vi "Calculate_Area_Difference_Short_Subtracks-1.vi"(4 "[IN] Areas particles\nPrimary Detected":dbl[][](array[numeric]), 5 "[IN] Start pos":i32, 6 "[IN] Primary \n(X,Y) Detected":dbl[][](array[numeric]), 7 "[IN] Subtrack":dbl[](array[numeric]), 8 "[IN] Index of \"11\" Dis-\nplacement in Subtrack":i32, 10 "[IN] Index of\n subtrack":i32, 11 "[IN] Areas \ndifference":dbl[](array[numeric])) -> (3 "[OUT] Areas \ndifference":dbl[](array[numeric]))   [LabVIEW 2013]
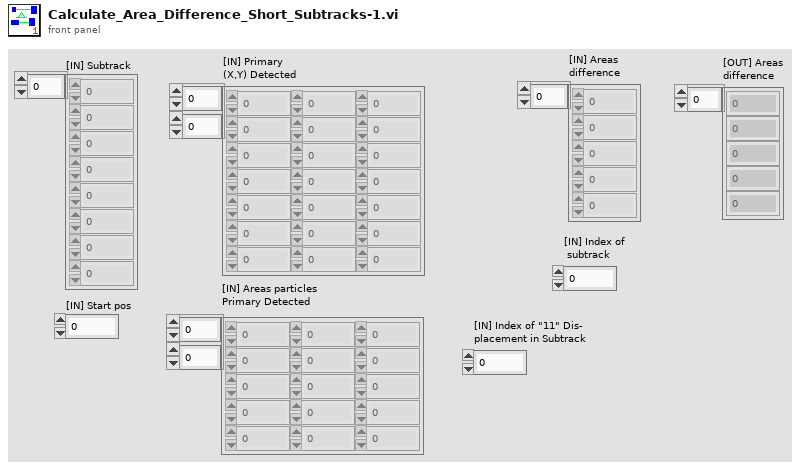
[diagram p1: front panel]
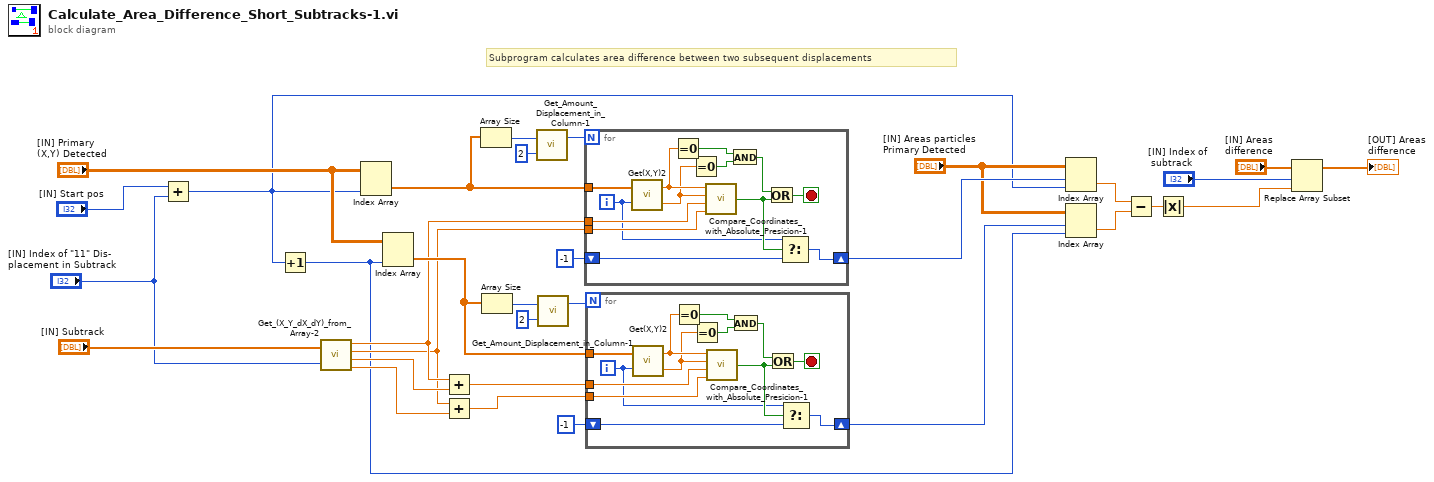
[diagram p0: block diagram]
diagram:
  # "Subprogram calculates area difference between two subsequent displacements"
  n1 = Add(x="[IN] Start pos", y="[IN] Index of \"11\" Dis-\nplacement in Subtrack") -> (x+y=w2:i32)
  n2 = Increment(x=w2) -> (x+1=w1:i32)
  n3 = call "Get_(X_Y_dX_dY)_from_Array-2.vi"("(X,Y,dX,dY)"="[IN] Subtrack", "Index of Displacement"="[IN] Index of \"11\" Dis-\nplacement in Subtrack") -> ("X"=w8:dbl, "Y"=w4:dbl, "dX"=w7:dbl, "dY"=w3:dbl)
  n4 = Index Array(array="[IN] Primary \n(X,Y) Detected", index (col)=w2) -> (element=w27:dbl[])  [unwired: 1 in]
  n5 = Index Array(array="[IN] Primary \n(X,Y) Detected", index (col)=w1) -> (element=w20:dbl[])  [unwired: 1 in]
  n6 = Add(x=w8, y=w7) -> (x+y=w6:dbl)
  n7 = Add(x=w4, y=w3) -> (x+y=w5:dbl)
  n8 = Array Size(array=w27) -> (size(s)=w31:i32)
  n9 = Array Size(array=w20) -> (size(s)=w26:i32)
  n10 = call "Get_Amount_Displacement_in_Column-1.vi"("multiplier"=2, "# Rows"=w31) -> ("Displ amount"=w29:i32)  [unwired: 1 out]
  n11 = call "Get_Amount_Displacement_in_Column-1.vi"("multiplier"=2, "# Rows"=w26) -> ("Displ amount"=w24:i32)  [unwired: 1 out]
  n12 = for {
    N: w29 -> [_]
    tunnel: w27 -> [w44]
    tunnel: w8 -> [w43]
    tunnel: w4 -> [w42]
    shift-right: [w33] -> w19
    shift-left: -1 -> [w34]
    i -> [w35]
    stop <- w45 stop-if-true
    n13 = call "Get(X,Y)2.vi"("[IN] index of (X,Y)"=w35, "[IN] Array coordi\nnates (X,Y) in Frame"=w44) -> ("[OUT] Y"=w38:dbl, "[OUT] X"=w39:dbl)
    n14 = Equal To 0?(x=w39) -> (x = 0?=w41:bool)
    n15 = Equal To 0?(x=w38) -> (x = 0?=w40:bool)
    n16 = call "Compare_Coordinates_with_Absolute_Presicion-1.vi"("X 1"=w39, "Y 1"=w38, "X 2"=w43, "Y 2"=w42) -> ("[OUT] Same coordinates?"=w36:bool)  [unwired: 1 in]
    n17 = And(x=w41, y=w40) -> (x .and. y?=w37:bool)
    n18 = Or(x=w37, y=w36) -> (x .or. y?=w45:bool)
    n19 = Select(t=w35, s=w36, f=w34) -> (s? t:f=w33:i32)
  }
  n20 = for {
    N: w24 -> [_]
    tunnel: w20 -> [w57]
    tunnel: w6 -> [w56]
    tunnel: w5 -> [w55]
    shift-right: [w46] -> w17
    shift-left: -1 -> [w47]
    i -> [w48]
    stop <- w58 stop-if-true
    n21 = call "Get(X,Y)2.vi"("[IN] index of (X,Y)"=w48, "[IN] Array coordi\nnates (X,Y) in Frame"=w57) -> ("[OUT] Y"=w51:dbl, "[OUT] X"=w52:dbl)
    n22 = Equal To 0?(x=w52) -> (x = 0?=w54:bool)
    n23 = Equal To 0?(x=w51) -> (x = 0?=w53:bool)
    n24 = call "Compare_Coordinates_with_Absolute_Presicion-1.vi"("X 1"=w52, "Y 1"=w51, "X 2"=w56, "Y 2"=w55) -> ("[OUT] Same coordinates?"=w49:bool)  [unwired: 1 in]
    n25 = And(x=w54, y=w53) -> (x .and. y?=w50:bool)
    n26 = Or(x=w50, y=w49) -> (x .or. y?=w58:bool)
    n27 = Select(t=w48, s=w49, f=w47) -> (s? t:f=w46:i32)
  }
  n28 = Index Array(array="[IN] Areas particles\nPrimary Detected", index (row)=w19, index (col)=w2) -> (element=w16:dbl)
  n29 = Index Array(array="[IN] Areas particles\nPrimary Detected", index (row)=w17, index (col)=w1) -> (element=w15:dbl)
  n30 = Subtract(x=w16, y=w15) -> (x-y=w14:dbl)
  n31 = Absolute Value(x=w14) -> (abs(x)=w11:dbl)
  n32 = Replace Array Subset(array="[IN] Areas \ndifference", new element=w11, index="[IN] Index of\n subtrack") -> (→"[OUT] Areas \ndifference":dbl[])
